vi "WPI_SolenoidCache.vi"(7 "AllocatedSolenoidOp":T2, 8 "error in (no error)":errorcluster, 10 "SolenoidChannel":T1=enum."Solenoid 1", 11 "Pneumatics Control Module":u8) -> (0 "error out":errorcluster, 2 "AllocatedSolenoidChannel":T1=enum."Solenoid 1", 3 "Allocated":bool)   [LabVIEW 2017]
doc: "This software is licensed. Open the labview\\readme\\WPI Robotics Library Open Source License.txt file for more information."
uses:
  <vilib>/Rock Robotics/WPI/Solenoid/WPI_SolenoidChannel.ctl
  <vilib>/Rock Robotics/WPI/Solenoid/WPI_SolenoidCacheOp.ctl
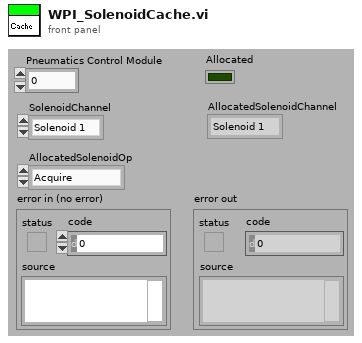
[diagram p1: front panel]
types:
  T1 = typedef "WPI_SolenoidChannel.ctl" = enum8{"Solenoid 0", "Solenoid 1", "Solenoid 2", "Solenoid 3", "Solenoid 4", "Solenoid 5", "Solenoid 6", "Solenoid 7", "Invalid"}
  T2 = typedef "WPI_SolenoidCacheOp.ctl" = enum16{"Acquire", "Release", "Status"}
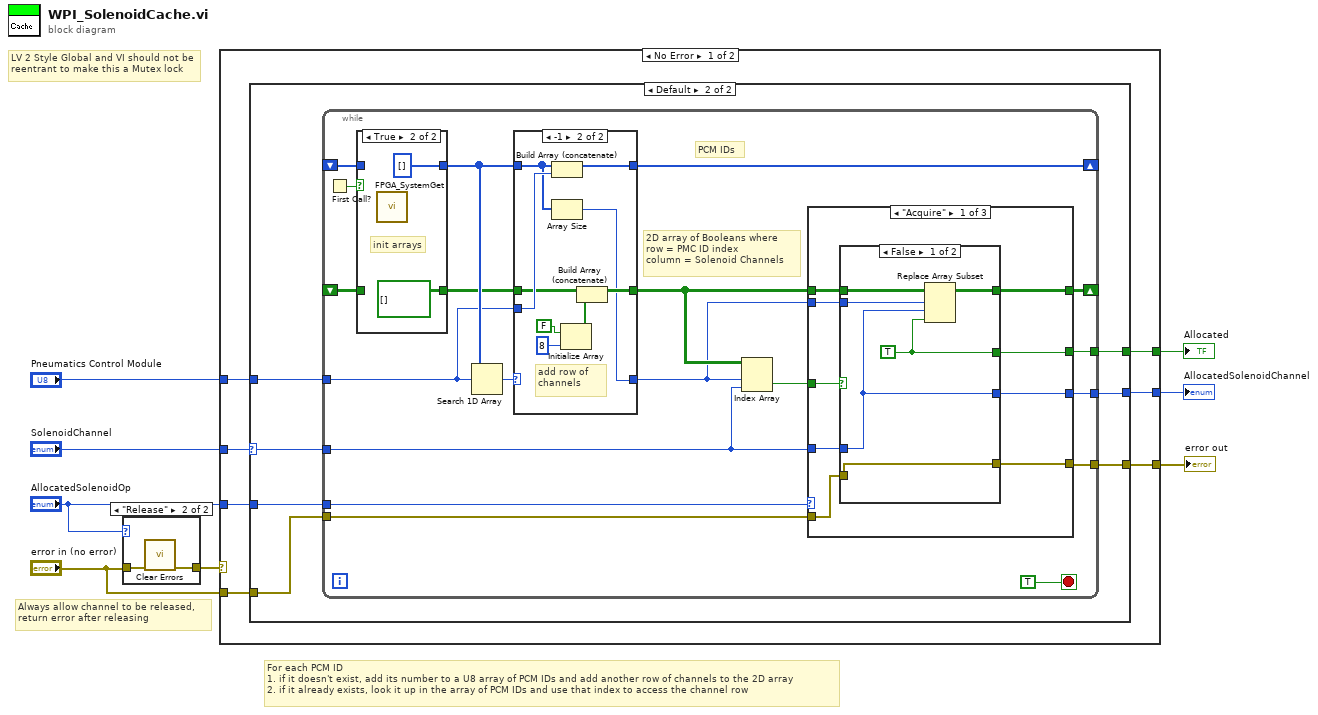
[diagram p0: block diagram]
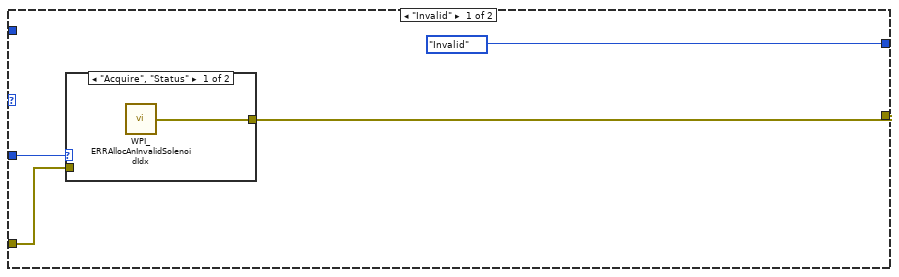
[diagram p2: hidden frame]
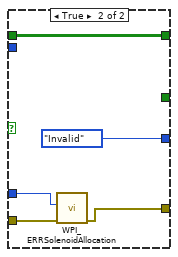
[diagram p4: hidden frame]
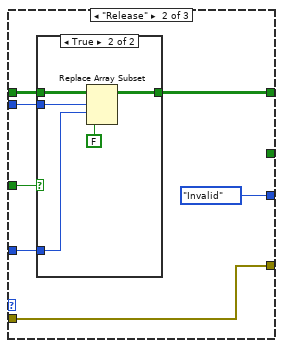
[diagram p5: hidden frame]
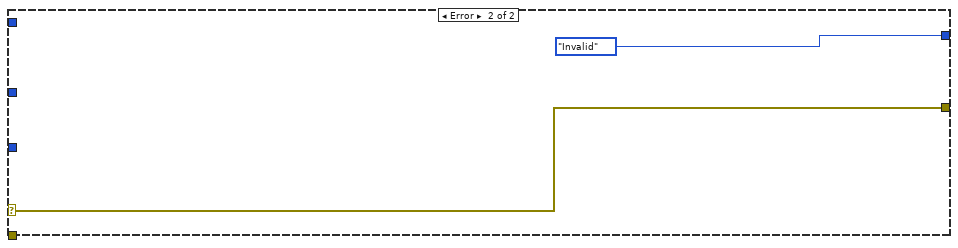
[diagram p10: hidden frame]
diagram:
  # "For each PCM ID\n1. if it doesn't exist, add its number to a U8 array of PCM IDs and add another row of channels to the 2D array\n2. if it already exists, look it up in the array of PCM IDs and use that index to access the channel row"
  # "LV 2 Style Global and VI should not be reentrant to make this a Mutex lock"
  # "Always allow channel to be released,\nreturn error after releasing"
  n1 = case shown="\"Release\"" "AllocatedSolenoidOp" {
    tunnel: "error in (no error)" -> [w9 w11]
    tunnel: [w9 w10] -> w6
    frame "Acquire", Default {
    }
    frame "Release" {
      n2 = call <vilib>:"Clear Errors.vi"("error in (no error)"=w11) -> ("error out"=w10:errorcluster)  [unwired: 1 in, 5 out]
    }
  }
  n3 = case shown="No Error" w6 {
    selector: w6 -> [_ w103]
    tunnel: "AllocatedSolenoidOp" -> [w18 _]
    tunnel: "SolenoidChannel" -> [w17 _]
    tunnel: [w16 w103] -> w1
    tunnel: [w15 _] -> w4
    tunnel: "Pneumatics Control Module" -> [w13 _]
    tunnel: [w14 WPI_SolenoidChannel."Invalid" ("AllocatedSolenoidChannel")] -> w3
    tunnel: "error in (no error)" -> [w12 _]
    frame No Error {
      n4 = case shown="Default" w17 {
        selector: w17 -> [_ w25]
        tunnel: w18 -> [w22 w30]
        tunnel: [w21 w29] -> w16
        tunnel: [_ w28] -> w15
        tunnel: w13 -> [_ w27]
        tunnel: [WPI_SolenoidChannel."Invalid" ("AllocatedSolenoidChannel") w26] -> w14
        tunnel: w12 -> [w19 w24]
        frame "Invalid" {
          n5 = case shown="\"Acquire\", \"Status\"" w22 {
            tunnel: [w23 _] -> w21
            tunnel: w19 -> [_ _]
            frame "Acquire", "Status" {
              n6 = call <vilib>:"WPI_ERRAllocAnInvalidSolenoidIdx.vi"() -> ("error out"=w23:errorcluster)
            }
            frame "Release" {
            }
          }
        }
        frame Default {
          n7 = while {
            shift-right: [w47] -> _
            shift-left: _ -> [w40]
            tunnel: w30 -> [w48]
            tunnel: w25 -> [w32]
            tunnel: [w46] -> w29
            tunnel: [w45] -> w28
            tunnel: w27 -> [w36]
            tunnel: [w43] -> w26
            tunnel: w24 -> [w42]
            shift-right: [w39] -> _
            shift-left: _ -> [w41]
            stop <- TRUE stop-if-true
            # "PCM IDs"
            # "2D array of Booleans where\nrow = PMC ID index\ncolumn = Solenoid Channels"
            n8 = First Call?() -> (First Call?: T/F=w49:bool)
            n9 = case shown="True" w49 {
              tunnel: [w100 u8[] []] -> w38
              tunnel: w41 -> [w100 _]
              tunnel: [w99 bool[][] []] -> w34
              tunnel: w40 -> [w99 _]
              frame False {
              }
              frame True {
                # "init arrays"
                n10 = call <vilib>:"FPGA_SystemGet.vi"() -> ()  [unwired: 2 in, 10 out]
              }
            }
            n11 = Search 1D Array(1D array=w38, element=w36) -> (index of element=w37:i32)  [unwired: 1 in]
            n12 = case shown="-1" w37 {
              selector: w37 -> [w87 _]
              tunnel: w38 -> [w89 w96]
              tunnel: [w89 w98] -> w39
              tunnel: w36 -> [_ w97]
              tunnel: w34 -> [w88 w95]
              tunnel: [w88 w94] -> w33
              tunnel: [w87 w90] -> w31
              frame Default {
              }
              frame -1 {
                # "add row of channels"
                n13 = Build Array (concatenate)(w96, w97) -> (w98:u8[])
                n14 = Array Size(array=w96) -> (size(s)=w90:i32)
                n15 = Initialize Array(FALSE, 8) -> (w91:bool[])
                n16 = Build Array (concatenate)(w95, w91) -> (w94:bool[][])
              }
            }
            n17 = Index Array(array=w33, index (row)=w31, index (col)=w32) -> (element=w35:bool)
            n18 = case shown="\"Acquire\"" w48 {
              tunnel: w33 -> [w54 w76 w85]
              tunnel: [w58 w74 w85] -> w47
              tunnel: w32 -> [w57 w75 w84]
              tunnel: [w56 w71 w83] -> w46
              tunnel: [w55 _ w86] -> w45
              tunnel: w35 -> [w53 w73 w86]
              tunnel: [w52 WPI_SolenoidChannel."Invalid" ("AllocatedSolenoidChannel") w84] -> w43
              tunnel: w42 -> [w50 w71 w83]
              tunnel: w31 -> [w51 w70 _]
              frame "Acquire" {
                n19 = case shown="False" w53 {
                  tunnel: w54 -> [w63 w69]
                  tunnel: [w62 w69] -> w58
                  tunnel: w57 -> [w60 w65]
                  tunnel: [w61 w67] -> w56
                  tunnel: [w64 _] -> w55
                  tunnel: [w60 WPI_SolenoidChannel."Invalid" ("AllocatedSolenoidChannel")] -> w52
                  tunnel: w50 -> [w61 w66]
                  tunnel: w51 -> [w59 _]
                  frame False {
                    w64 = TRUE ("new element/subarray")
                    n20 = Replace Array Subset(array=w63, new element=w64, index (row)=w59, index (col)=w60) -> (w62:bool[][])
                  }
                  frame True {
                    n21 = call <vilib>:"WPI_ERRSolenoidAllocation.vi"("error in (no error)"=w66, "SolenoidChannel"=w65) -> ("ERRSolenoidAllocation"=w67:errorcluster)  [unwired: 9 in]
                  }
                }
              }
              frame "Release" {
                n22 = case shown="True" w73 {
                  tunnel: w76 -> [w77 w82]
                  tunnel: w75 -> [_ w79]
                  tunnel: [w77 w81] -> w74
                  tunnel: w70 -> [_ w78]
                  frame False {
                  }
                  frame True {
                    n23 = Replace Array Subset(array=w82, new element=FALSE ("new element/subarray"), index (row)=w78, index (col)=w79) -> (w81:bool[][])
                  }
                }
              }
              frame "Status" {
              }
            }
          }
        }
      }
    }
    frame Error {
    }
  }
  "Allocated" <- w4
  "error out" <- w1
  "AllocatedSolenoidChannel" <- w3
